vi "Units_MetersToInches.vi"(10 "Meters":dbl) -> (2 "Inches":dbl)   [LabVIEW 2019, in "Trajectory_Library.lvlib"]
doc: "Convert a value from meters to inches\n\nInputs: \n - Meters - Distance (Meters)\n\nOutputs:\n - Inches - Distance (Inches)"
uses:
  Trajectory_Library.lvlib
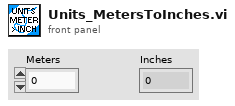
[diagram p1: front panel]
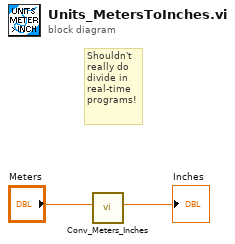
[diagram p0: block diagram]
diagram:
  # "Shouldn't\nreally do\ndivide in\nreal-time\nprograms!"
  n1 = call "Conv_Meters_Inches.vi"("Meters"="Meters") -> ("Inches"=→"Inches":dbl)  [unwired: 10 in]
